vi "32xx_Wr_Rd_String.vi"(6 "Attente avant lecture (ms)":u32=25, 7 "TimeOut (mS)":u32=6000, 8 "entrée d'erreur":errorcluster={"status"=FALSE, "code"=0, "source"="L'opération  de lecture s'est déroulée avec succès."}, 10 "String In":string="0 VOLT2 MES\r" caption="Chaîne à écrire", 11 "Visa In":refnum<visa-resource-name>="COM3" caption="Port d'entrée") -> (0 "sortie d'erreur":errorcluster={"status"=FALSE, "code"=0, "source"="L'opération  de lecture s'est déroulée avec succès."}, 2 "Réponse":string="0 OK 12021\r", 3 "Visa Out":refnum<visa-resource-name>="COM3" caption="Port de sortie", 4 "octets lus":u32=11, 5 "Acknowledge":bool=TRUE caption="'OK' reçu")   [LabVIEW 2020]
doc: "Écriture d'une commande sous forme de chaîne.\n& lecture de la réponse sous la même forme."
panel:
  # "© 2020 elc CORPORATION.  \nALL RIGHTS RESERVED."
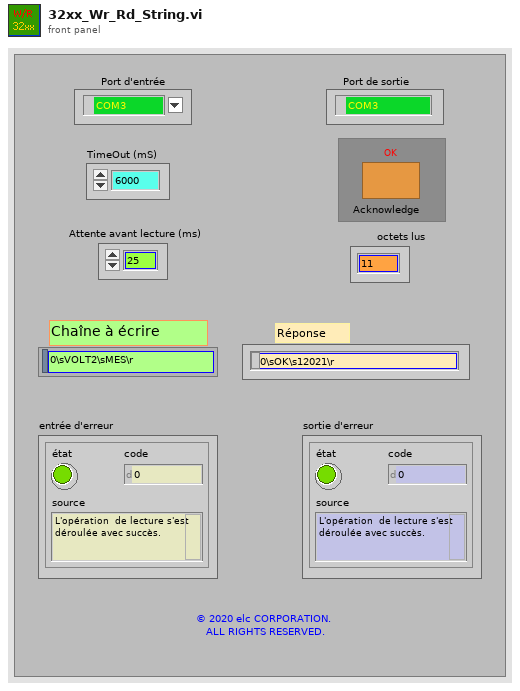
[diagram p1: front panel]
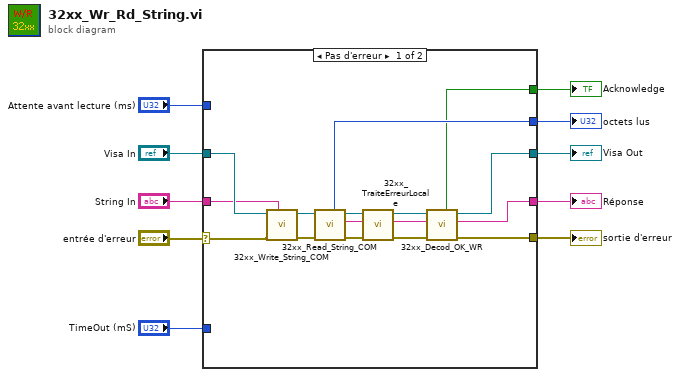
[diagram p0: block diagram]
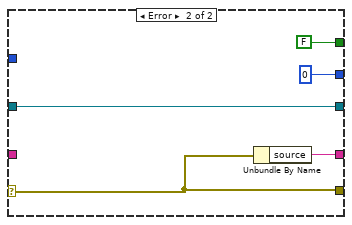
[diagram p2: hidden frame]
diagram:
  n1 = case shown="Pas d'erreur" "entrée d'erreur" {
    selector: "entrée d'erreur" -> [w25 w29]
    tunnel: [w12 w31] -> w10
    tunnel: [w14 w29] -> w9
    tunnel: "String In" -> [w24 _]
    tunnel: "Visa In" -> [w26 w31]
    tunnel: "Attente avant lecture (ms)" -> [_ _]
    tunnel: [w21 u32 0 ("octets lus")] -> w5
    tunnel: [w13 w30] -> w4
    tunnel: [w11 FALSE ("Acknowledge")] -> w3
    tunnel: "TimeOut (mS)" -> [_ _]
    frame No Error {
      n2 = call "32xx_Write_String_COM.vi"("Chaîne à écrire"=w24, "entrée d'erreur"=w25, "Port d'entrée"=w26) -> ("sortie d'erreur"=w22:errorcluster, "Port de sortie"=w23:refnum<visa-resource-name>)  [unwired: 7 in]
      n3 = call "32xx_Read_String_COM.vi"("entrée d'erreur"=w22, "Port d'entrée"=w23) -> ("Sortie d'erreur"=w18:errorcluster, "Réponse"=w19:string, "Port de sortie"=w20:refnum<visa-resource-name>, "octets lus"=w21:u32)  [unwired: 6 in]
      n4 = call "32xx_TraiteErreurLocale.vi"("Entrée \nd'erreur"=w18, "Chaîne\nd'entrée"=w19, "Port d'entrée"=w20) -> ("Sortie \nd'erreur"=w15:errorcluster, "Chaîne de\nsortie"=w16:string, "Port de sortie"=w17:refnum<visa-resource-name>)  [unwired: 6 in]
      n5 = call "32xx_Decod_OK_WR.vi"("entrée d'erreur"=w15, "Entrée Chaîne Caractères"=w16, "Visa In"=w17) -> ("sortie d'erreur"=w14:errorcluster, "Sortie Chaîne Caractères"=w13:string, "Visa Out"=w12:refnum<visa-resource-name>, "Acknowledge"=w11:bool)  [unwired: 5 in]
    }
    frame Error {
      n6 = Unbundle By Name(w29) -> ("source"=w30:string)
    }
  }
  "Réponse" <- w4
  "octets lus" <- w5
  "sortie d'erreur" <- w9
  "Visa Out" <- w10
  "Acknowledge" <- w3
